vi "DMSO_transfer_sample_add_NaOH_reload_MQ_NaCl_subVI.vi"(0 "Extra Milli-Q (ml)":dbl=4.0, 1 "Pump Parameters":T1={"Speed 1"="100", "Speed 2"="250", "Speed 3"="250", "Speed 4"="250", "UW/Sample"="5", "Sparge"="2", "Std"="4", "Waste"="15", "Air"="14", "Milli-Q"="1", "H2SO4"="6", "NaOH"="3", "Catalyst"="7", "Cell (H+ side)"="8", "Cell (sample side)"="9", "NaCl"="9"}, 2 "Total Vol. (mL)":dbl, 3 "Reverse Reduction?":bool, 5 "Sample Vol. (mL)":dbl, 9 "step to ml":dbl=1920.0, 11 "NaOH Vol (mL)":dbl, 12 "Split DMSP sample?":bool, 13 "Remove DMSP vol. (mL)":dbl=4.0, 14 "COM Port":refnum<visa-resource-name>="COM7") -> ()   [LabVIEW 2021]
panel:
  out "Full Command":string="V100O1P7680O9D7680"
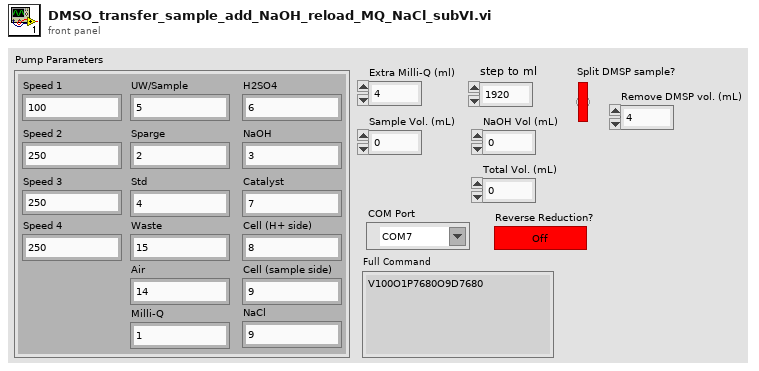
[diagram p1: front panel]
types:
  T1 = cluster{"Speed 1":string, "Speed 2":string, "Speed 3":string, "Speed 4":string, "UW/Sample":string, "Sparge":string, "Std":string, "Waste":string, "Air":string, "Milli-Q":string, "H2SO4":string, "NaOH":string, "Catalyst":string, "Cell (H+ side)":string, "Cell (sample side)":string, "NaCl":string}
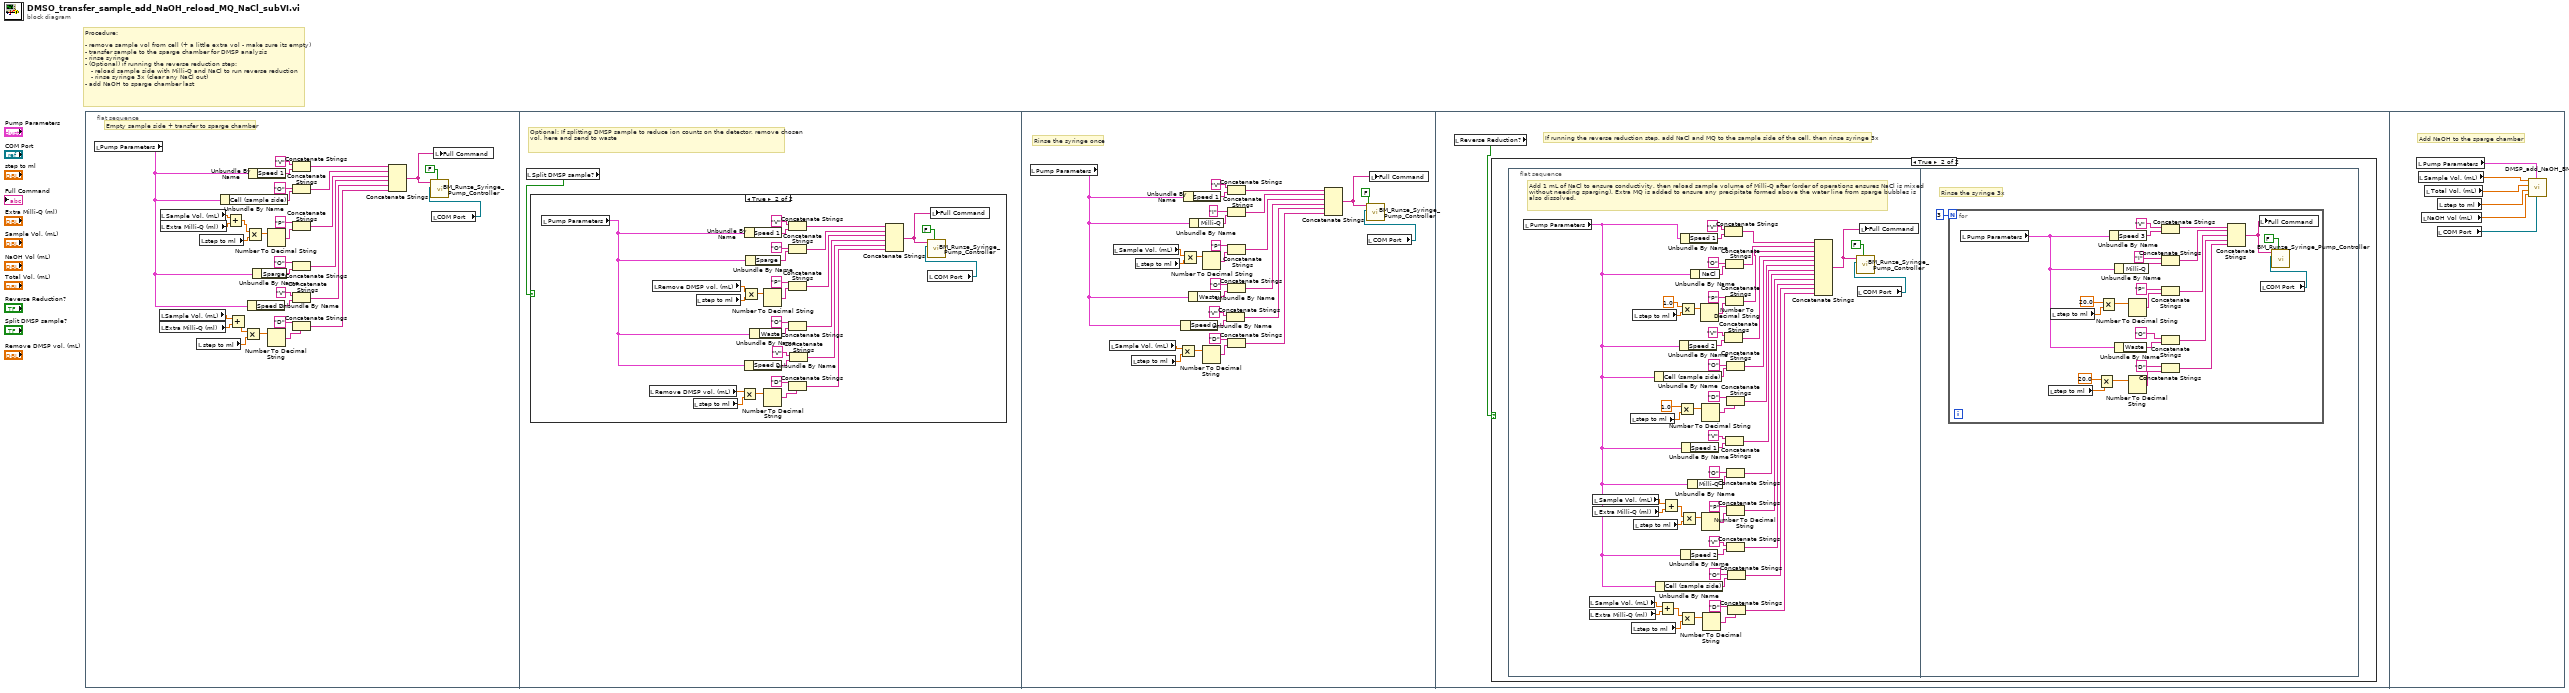
[diagram p0: block diagram]
diagram:
  # "Procedure:\n\n- remove sample vol from cell (+ a little extra vol - make sure its empty)\n- transfer sample to the sparge chamber for DMSP analysis\n- rinse syringe\n- (Optional) if running the reverse reduction step:\n   - reload sample side with Milli-Q and NaCl to run reverse reduction\n   - rinse syringe 3x (clear any NaCl out)\n- add NaOH to sparge chamber last"
  n1 = flat-sequence {
    frame #0 {
      # "Empty sample side + transfer to sparge chamber"
      n2 = local read "Pump Parameters"() -> (w10:T1)
      n3 = local read "Sample Vol. (mL)"() -> (w3:dbl)
      n4 = local read "Extra Milli-Q (ml)"() -> (w2:dbl)
      n5 = local read "Sample Vol. (mL)"() -> (w6:dbl)
      n6 = local read "Extra Milli-Q (ml)"() -> (w5:dbl)
      n7 = local read "step to ml"() -> (w23:dbl)
      n8 = local read "step to ml"() -> (w28:dbl)
      n9 = Unbundle By Name(w10) -> ("Cell (sample side)"=w8:string)
      n10 = Add(x=w6, y=w5) -> (x+y=w4:dbl)
      n11 = Add(x=w3, y=w2) -> (x+y=w1:dbl)
      n12 = Multiply(x=w1, y=w23) -> (x*y=w24:dbl)
      n13 = Multiply(x=w4, y=w28) -> (x*y=w29:dbl)
      n14 = Unbundle By Name(w10) -> ("Speed 2"=w13:string)
      n15 = Unbundle By Name(w10) -> ("Speed 1"=w30:string)
      n16 = Unbundle By Name(w10) -> ("Sparge"=w7:string)
      n17 = Number To Decimal String(number=w29) -> (decimal integer string=w26:string)  [unwired: 1 out]
      n18 = Number To Decimal String(number=w24) -> (decimal integer string=w21:string)  [unwired: 1 out]
      n19 = Concatenate Strings("V", w30) -> (w20:string)
      n20 = Concatenate Strings("O", w8) -> (w19:string)
      n21 = Concatenate Strings("P", w26) -> (w18:string)
      n22 = Concatenate Strings("O", w7) -> (w17:string)
      n23 = Concatenate Strings("D", w21) -> (w11:string)
      n24 = Concatenate Strings("V", w13) -> (w12:string)
      n25 = Concatenate Strings(w20, w19, w18, w17, w12, w11) -> (w16:string)
      n26 = local read "COM Port"() -> (w15:refnum<visa-resource-name>)
      n27 = call "BM_Runze_Syringe_Pump_Controller.vi"("Initialize Plunger?"=FALSE ("Initialize?"), "COM Port (Runze)"=w15, "Enter Command"=w16) -> ()  [unwired: 6 in, 3 out]
      n28 = local write "Full Command"(w16) -> ()
    }
    frame #1 {
      # "Optional: If splitting DMSP sample to reduce ion counts on the detector, remove chosen vol. here and send to waste"
      n29 = local read "Split DMSP sample?"() -> (w33:bool)
      n30 = case shown="True" w33 {
        frame False {
          # "If not splitting sample, continue with analysis"
        }
        frame True {
          n31 = local read "Pump Parameters"() -> (w45:T1)
          n32 = local read "Remove DMSP vol. (mL)"() -> (w35:dbl)
          n33 = local read "Remove DMSP vol. (mL)"() -> (w34:dbl)
          n34 = local read "step to ml"() -> (w56:dbl)
          n35 = local read "step to ml"() -> (w59:dbl)
          n36 = Multiply(x=w35, y=w56) -> (x*y=w57:dbl)
          n37 = Multiply(x=w34, y=w59) -> (x*y=w60:dbl)
          n38 = Unbundle By Name(w45) -> ("Speed 2"=w48:string)
          n39 = Unbundle By Name(w45) -> ("Speed 1"=w61:string)
          n40 = Unbundle By Name(w45) -> ("Sparge"=w44:string)
          n41 = Unbundle By Name(w45) -> ("Waste"=w43:string)
          n42 = Number To Decimal String(number=w60) -> (decimal integer string=w58:string)  [unwired: 1 out]
          n43 = Number To Decimal String(number=w57) -> (decimal integer string=w55:string)  [unwired: 1 out]
          n44 = Concatenate Strings("V", w61) -> (w54:string)
          n45 = Concatenate Strings("O", w44) -> (w53:string)
          n46 = Concatenate Strings("P", w58) -> (w52:string)
          n47 = Concatenate Strings("O", w43) -> (w51:string)
          n48 = Concatenate Strings("D", w55) -> (w46:string)
          n49 = Concatenate Strings("V", w48) -> (w47:string)
          n50 = Concatenate Strings(w54, w53, w52, w51, w47, w46) -> (w50:string)
          n51 = local read "COM Port"() -> (w49:refnum<visa-resource-name>)
          n52 = call "BM_Runze_Syringe_Pump_Controller.vi"("Initialize Plunger?"=FALSE ("Initialize?"), "COM Port (Runze)"=w49, "Enter Command"=w50) -> ()  [unwired: 6 in, 3 out]
          n53 = local write "Full Command"(w50) -> ()
        }
      }
    }
    frame #2 {
      # "Rinse the syringe once"
      n54 = local read "Pump Parameters"() -> (w89:T1)
      n55 = local read "Sample Vol. (mL)"() -> (w81:dbl)
      n56 = local read "Sample Vol. (mL)"() -> (w78:dbl)
      n57 = local read "step to ml"() -> (w83:dbl)
      n58 = local read "step to ml"() -> (w75:dbl)
      n59 = Multiply(x=w81, y=w83) -> (x*y=w82:dbl)
      n60 = Unbundle By Name(w89) -> ("Speed 2"=w85:string)
      n61 = Multiply(x=w78, y=w75) -> (x*y=w76:dbl)
      n62 = Unbundle By Name(w89) -> ("Speed 1"=w77:string)
      n63 = Unbundle By Name(w89) -> ("Waste"=w80:string)
      n64 = Unbundle By Name(w89) -> ("Milli-Q"=w79:string)
      n65 = Number To Decimal String(number=w82) -> (decimal integer string=w84:string)  [unwired: 1 out]
      n66 = Number To Decimal String(number=w76) -> (decimal integer string=w74:string)  [unwired: 1 out]
      n67 = Concatenate Strings("V", w85) -> (w87:string)
      n68 = Concatenate Strings("D", w84) -> (w88:string)
      n69 = Concatenate Strings("V", w77) -> (w73:string)
      n70 = Concatenate Strings("I", w79) -> (w72:string)
      n71 = Concatenate Strings("P", w74) -> (w71:string)
      n72 = Concatenate Strings("O", w80) -> (w86:string)
      n73 = Concatenate Strings(w73, w72, w71, w86, w87, w88) -> (w70:string)
      n74 = local read "COM Port"() -> (w69:refnum<visa-resource-name>)
      n75 = call "BM_Runze_Syringe_Pump_Controller.vi"("Initialize Plunger?"=FALSE ("Initialize?"), "COM Port (Runze)"=w69, "Enter Command"=w70) -> ()  [unwired: 6 in, 3 out]
      n76 = local write "Full Command"(w70) -> ()
    }
    frame #3 {
      # "If running the reverse reduction step, add NaCl and MQ to the sample side of the cell, then rinse syringe 3x"
      n77 = local read "Reverse Reduction?"() -> (w90:bool)
      n78 = case shown="True" w90 {
        frame False {
        }
        frame True {
          n79 = flat-sequence {
            frame #0 {
              # "Add 1 mL of NaCl to ensure conductivity, then reload sample volume of Milli-Q after (order of operations ensures NaCl is mixed without needing sparging). Extra MQ is added to ensure any precipitate formed above the water line from sparge bubbles is also dissolved."
              n80 = local read "Pump Parameters"() -> (w109:T1)
              n81 = local read "Sample Vol. (mL)"() -> (w93:dbl)
              n82 = local read "Extra Milli-Q (ml)"() -> (w94:dbl)
              n83 = local read "Sample Vol. (mL)"() -> (w96:dbl)
              n84 = local read "Extra Milli-Q (ml)"() -> (w95:dbl)
              n85 = local read "step to ml"() -> (w134:dbl)
              n86 = local read "step to ml"() -> (w125:dbl)
              n87 = local read "step to ml"() -> (w141:dbl)
              n88 = local read "step to ml"() -> (w118:dbl)
              n89 = Unbundle By Name(w109) -> ("Cell (sample side)"=w136:string)
              n90 = Unbundle By Name(w109) -> ("Cell (sample side)"=w123:string)
              n91 = Add(x=w93, y=w94) -> (x+y=w91:dbl)
              n92 = Add(x=w96, y=w95) -> (x+y=w92:dbl)
              n93 = Multiply(x=1.0, y=w134) -> (x*y=w135:dbl)
              n94 = Multiply(x=1.0, y=w141) -> (x*y=w142:dbl)
              n95 = Multiply(x=w91, y=w125) -> (x*y=w124:dbl)
              n96 = Unbundle By Name(w109) -> ("Speed 2"=w130:string)
              n97 = Unbundle By Name(w109) -> ("Speed 1"=w138:string)
              n98 = Multiply(x=w92, y=w118) -> (x*y=w117:dbl)
              n99 = Unbundle By Name(w109) -> ("Speed 2"=w129:string)
              n100 = Unbundle By Name(w109) -> ("Speed 1"=w121:string)
              n101 = Unbundle By Name(w109) -> ("Milli-Q"=w115:string)
              n102 = Unbundle By Name(w109) -> ("NaCl"=w145:string)
              n103 = Number To Decimal String(number=w142) -> (decimal integer string=w139:string)  [unwired: 1 out]
              n104 = Number To Decimal String(number=w135) -> (decimal integer string=w132:string)  [unwired: 1 out]
              n105 = Number To Decimal String(number=w117) -> (decimal integer string=w120:string)  [unwired: 1 out]
              n106 = Number To Decimal String(number=w124) -> (decimal integer string=w127:string)  [unwired: 1 out]
              n107 = Concatenate Strings("V", w138) -> (w108:string)
              n108 = Concatenate Strings("V", w130) -> (w105:string)
              n109 = Concatenate Strings("O", w145) -> (w107:string)
              n110 = Concatenate Strings("P", w139) -> (w106:string)
              n111 = Concatenate Strings("V", w121) -> (w102:string)
              n112 = Concatenate Strings("O", w136) -> (w104:string)
              n113 = Concatenate Strings("D", w132) -> (w103:string)
              n114 = Concatenate Strings("V", w129) -> (w99:string)
              n115 = Concatenate Strings("O", w115) -> (w101:string)
              n116 = Concatenate Strings("P", w120) -> (w100:string)
              n117 = Concatenate Strings("O", w123) -> (w98:string)
              n118 = Concatenate Strings("D", w127) -> (w97:string)
              n119 = Concatenate Strings(w108, w107, w106, w105, w104, w103, w102, w101, w100, w99, w98, w97) -> (w114:string)
              n120 = local read "COM Port"() -> (w113:refnum<visa-resource-name>)
              n121 = call "BM_Runze_Syringe_Pump_Controller.vi"("Initialize Plunger?"=FALSE ("Initialize?"), "COM Port (Runze)"=w113, "Enter Command"=w114) -> ()  [unwired: 6 in, 3 out]
              n122 = local write "Full Command"(w114) -> ()
            }
            frame #1 {
              # "Rinse the syringe 3x"
              n123 = for {
                N: 3 -> [_]
                n124 = local read "Pump Parameters"() -> (w154:T1)
                n125 = local read "step to ml"() -> (w155:dbl)
                n126 = local read "step to ml"() -> (w166:dbl)
                n127 = Multiply(x=20.0, y=w155) -> (x*y=w158:dbl)
                n128 = Multiply(x=20.0, y=w166) -> (x*y=w167:dbl)
                n129 = Unbundle By Name(w154) -> ("Speed 3"=w162:string)
                n130 = Unbundle By Name(w154) -> ("Milli-Q"=w169:string)
                n131 = Unbundle By Name(w154) -> ("Waste"=w160:string)
                n132 = Number To Decimal String(number=w167) -> (decimal integer string=w164:string)  [unwired: 1 out]
                n133 = Number To Decimal String(number=w158) -> (decimal integer string=w157:string)  [unwired: 1 out]
                n134 = Concatenate Strings("V", w162) -> (w153:string)
                n135 = Concatenate Strings("I", w169) -> (w152:string)
                n136 = Concatenate Strings("P" ("string"), w164) -> (w151:string)
                n137 = Concatenate Strings("O", w160) -> (w150:string)
                n138 = Concatenate Strings("D" ("string"), w157) -> (w149:string)
                n139 = Concatenate Strings(w153, w152, w151, w150, w149) -> (w170:string)
                n140 = local write "Full Command"(w170) -> ()
                n141 = local read "COM Port"() -> (w171:refnum<visa-resource-name>)
                n142 = call "BM_Runze_Syringe_Pump_Controller.vi"("Initialize Plunger?"=FALSE ("Initialize?"), "COM Port (Runze)"=w171, "Enter Command"=w170) -> ()  [unwired: 6 in, 3 out]
              }
            }
          }
        }
      }
    }
    frame #4 {
      # "Add NaOH to the sparge chamber"
      n143 = local read "Pump Parameters"() -> (w177:T1)
      n144 = local read "Sample Vol. (mL)"() -> (w176:dbl)
      n145 = local read "NaOH Vol (mL)"() -> (w173:dbl)
      n146 = local read "Total Vol. (mL)"() -> (w175:dbl)
      n147 = local read "COM Port"() -> (w178:refnum<visa-resource-name>)
      n148 = local read "step to ml"() -> (w174:dbl)
      n149 = call "DMSP_add_NaOH_BM.vi"("COM Port"=w178, "Pump Parameters"=w177, "NaOH Vol (mL)"=w173, "step to ml"=w174, "Total Vol. (mL)"=w175, "Sample Vol. (mL)"=w176) -> ()  [unwired: 6 in]
    }
  }
